vi "Ch4DIY.vi"() -> ()   [LabVIEW 2015]
panel:
  in  "stop":bool
  in  "Boolean":bool
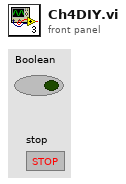
[diagram p1: front panel]
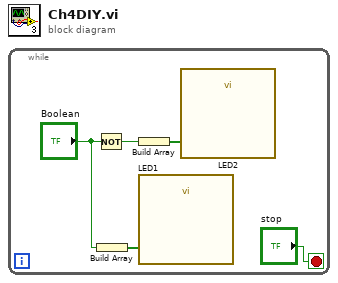
[diagram p0: block diagram]
diagram:
  n1 = while {
    stop <- "stop" stop-if-true
    n2 = Not(x="Boolean") -> (.not. x?=w2:bool)
    n3 = Build Array("Boolean") -> (w4:bool[])
    n4 = Build Array(w2) -> (w1:bool[])
    n5 = call "LED1"("data"=w4) -> ()  [unwired: 17 in, 2 out]
    n6 = call "LED2"("data"=w1) -> ()  [unwired: 17 in, 2 out]
  }
